vi "Head.vi"(0 "Boolean IN":bool, 13 "Slide":dbl(slide) scale=0.0..10.0) -> (20 "Boolean OUT":bool)   [LabVIEW 2025]
panel:
  out "Boolean":bool
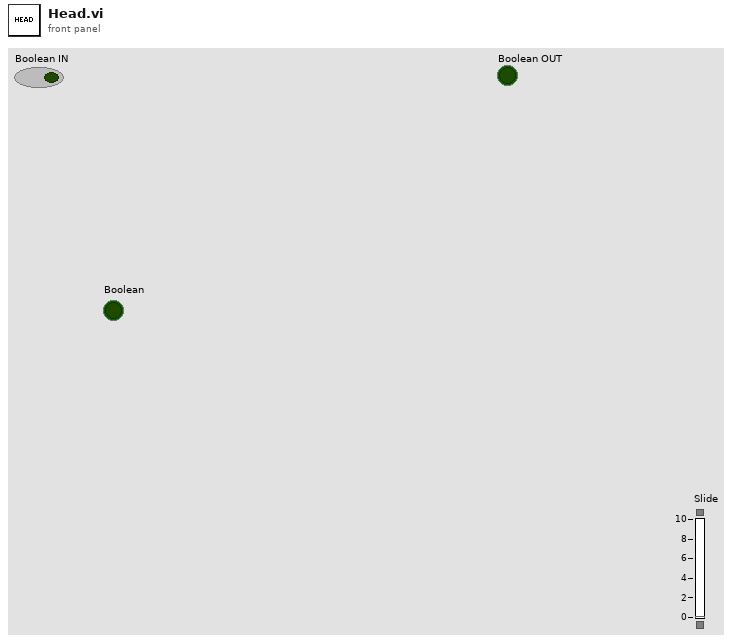
[diagram p1: front panel]
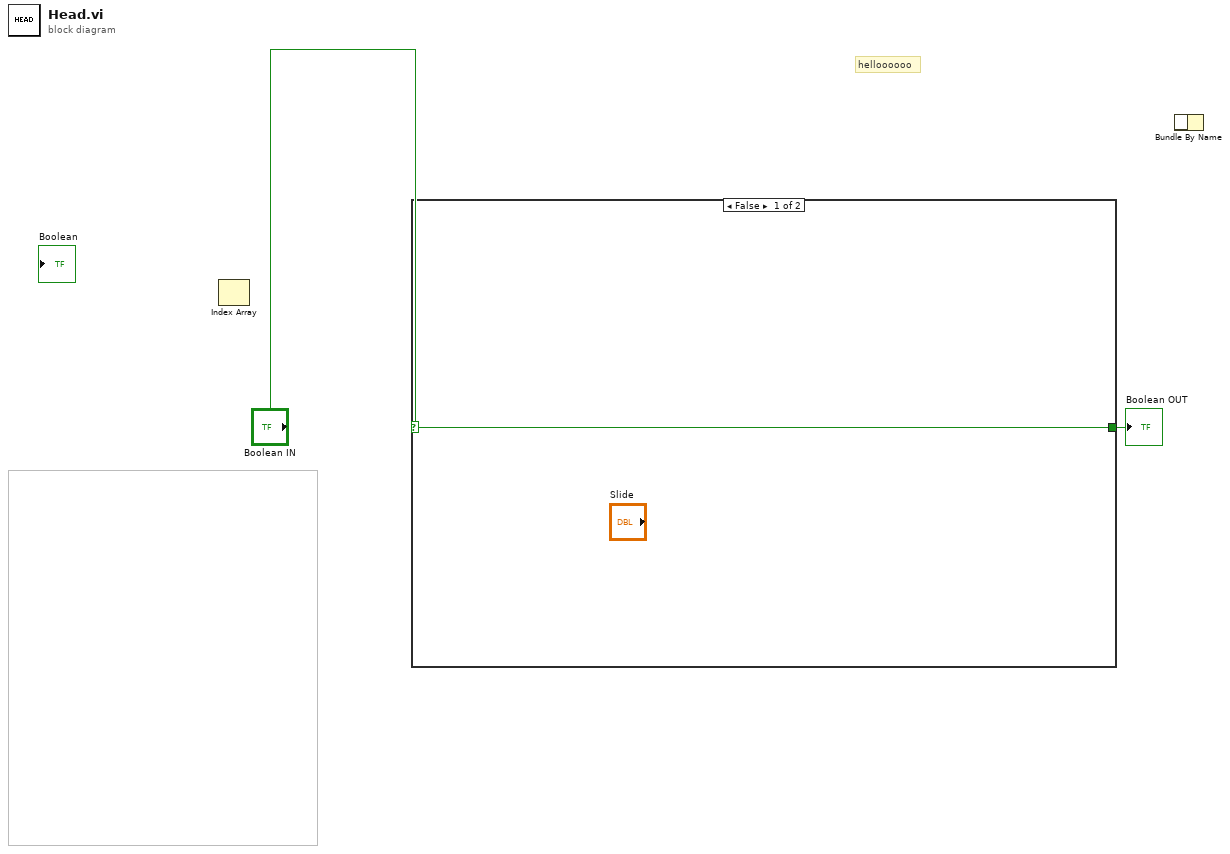
[diagram p0: block diagram]
diagram:
  # "helloooooo"
  n1 = Index Array() -> ()  [unwired: 2 in, 1 out]
  n2 = case shown="False" "Boolean IN" {
    selector: "Boolean IN" -> [w3 w4]
    tunnel: [w3 w4] -> w1
    frame False {
    }
    frame True {
    }
  }
  "Boolean OUT" <- w1
  n3 = Bundle By Name() -> ()  [unwired: 2 in, 1 out]
